vi "create.TradeExpanded.vi"(8 "error in (no error)":errorcluster, 11 "TradeExpanded.Parmeters":T1={"Time Offset"=447000, "Order Id"="ORID0001", "Side Indicator"="B", "Quantity"=20000, "Symbol"="AAPL", "Price"=0.905, "Execution Id"="EXE_ID_1"}) -> (0 "error out":errorcluster, 2 "Bytes.out":u8[](array[numeric]) format="%.0x", 3 "MessageBase out":refnum<class "TradeExpanded.lvclass">)   [LabVIEW 2022 SP3]
uses:
  Trade/TradeExpanded.Parameters.ctl
  Trade/TradeExpanded.lvclass
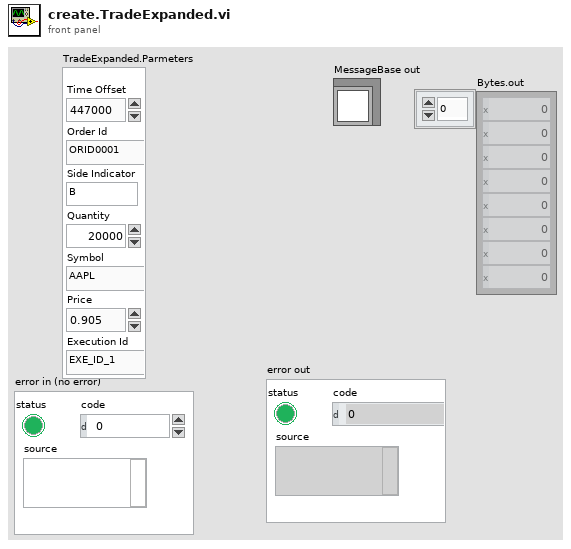
[diagram p1: front panel]
types:
  T1 = typedef "TradeExpanded.lvclass/TradeExpanded.Parameters.ctl" = cluster{"Time Offset":u32, "Order Id":string, "Side Indicator":string, "Quantity":u32, "Symbol":string, "Price":dbl, "Execution Id":string}
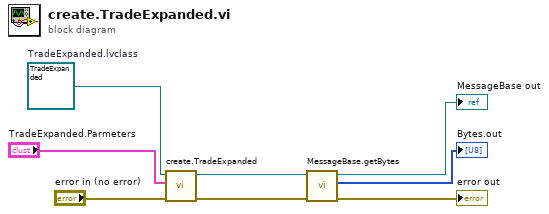
[diagram p0: block diagram]
diagram:
  w6 = refnum<class "TradeExpanded.lvclass"> refnum  # TradeExpanded.lvclass
  n1 = call-dynamic "create.TradeExpanded.vi"("error in"="error in (no error)", "TradeExpanded.Parameters"="TradeExpanded.Parmeters", "TradeExpanded in"=w6) -> ("error out"=w3:errorcluster, "TradeExpanded out"=w2:refnum<class "TradeExpanded.lvclass">)  [unwired: 7 in]
  n2 = call-dynamic "MessageBase.getBytes.vi"("error in (no error)"=w3, "MessageBase in"=w2) -> ("error out"=→"error out":errorcluster, "Bytes.out"=→"Bytes.out":u8[], "MessageBase out"=→"MessageBase out":refnum<class "TradeExpanded.lvclass">)  [unwired: 7 in]
